vi "Table Size with and without Results.vi"(8 "error in":errorcluster, 9 "Table Configuration (Eingang)":T8 {"Cell Defaults"."Vertical Align" items=["Bottom", "Middle", "Top"]; "Cell Defaults"."Horizontal Align" items=["Center", "Justified", "JustifiedAll", "Left", "Right"]; "Table Settings"."Horizontal Align" items=["Center"=0, "Left"=3, "Right"=4]}, 11 "Table Content":T3={"TableHeader"=["Soll\nppm/%", "Ist\nppm/%", "Fehler\n%", "Toleranz\n%", "Ergebnis"], "Table"=[], "Relative Column Widths (%)"=[], "Results"={"Results"=[], "ResultPictures"={"Yes Ctl Refnum"=refnum, "No Ctl Refnum"=refnum}, "use Pictures"=FALSE, "Image Scale (%)"=100.0, "Autoscale? (T)"=TRUE, "Horizontal Align"=3, "Position"=0}, "PositionBemerkung"=enum."before", "PageBreak"=enum."before", "TablePictures"={"Ctl Refnum In"=[], "RowOrColumn"=enum."Row", "IndexToInsert"=0, "Image Scale (%)"=[], "Autoscale? (T)"=[], "Horizontal Align"=3}, "Horizontal Align"=3} {"Horizontal Align" items=["Center", "Justified", "JustifiedAll", "Left", "Right"]; "TablePictures"."Horizontal Align" items=["Center", "Justified", "JustifiedAll", "Left", "Right"]; "Results"."Position" items=["First", "Last"]; "Results"."Horizontal Align" items=["Center", "Justified", "JustifiedAll", "Left", "Right"]}) -> (0 "error out":errorcluster, 1 "Table Configuration (Ausgang)":T8 {"Cell Defaults"."Vertical Align" items=["Bottom", "Middle", "Top"]; "Cell Defaults"."Horizontal Align" items=["Center", "Justified", "JustifiedAll", "Left", "Right"]; "Table Settings"."Horizontal Align" items=["Center"=0, "Left"=3, "Right"=4]}, 2 "Table out":string[][](array[string]), 3 "Results out":T4={"Results"=[], "ResultPictures"={"Yes Ctl Refnum"=refnum, "No Ctl Refnum"=refnum}, "use Pictures"=FALSE, "Image Scale (%)"=100.0, "Autoscale? (T)"=TRUE, "Horizontal Align"=3, "Position"=0} {"Position" items=["First", "Last"]; "Horizontal Align" items=["Center", "Justified", "JustifiedAll", "Left", "Right"]}, 4 "Empty-Cluster":T1, 5 "TablePictures out":T2={"Ctl Refnum In"=[], "RowOrColumn"=enum."Row", "IndexToInsert"=0, "Image Scale (%)"=[], "Autoscale? (T)"=[], "Horizontal Align"=3} {"Horizontal Align" items=["Center", "Justified", "JustifiedAll", "Left", "Right"]}, 6 "TableHeader out":string[](array[string]), 7 "Horizontal Align":i32)   [LabVIEW 2020, in "PDF Interface.lvlib" / "PDF Interface Helper.lvlib"]
uses:
  PDF Interface Helper.lvlib
  <vilib>/Simplicity AI/SAI_PDF_API/Classes/Table Builder/Controls/SAI_PDF_Table Configuration.ctl
  <vilib>/Simplicity AI/SAI_PDF_API/Classes/Table Builder/Controls/SAI_PDF_Table Horizontal Align.ctl
  <vilib>/Simplicity AI/SAI_PDF_API/Classes/Table Builder/Controls/SAI_PDF_Default Cell Format.ctl
  <vilib>/Simplicity AI/SAI_PDF_API/Classes/Table Builder/Controls/SAI_PDF_BorderLine.ctl
  PDFResults.ctl
  PDFResultPictures.ctl
  PDFTableContentType.ctl
  PDFCommentPosition.ctl
  PDFPageBreak.ctl
  PDFTablePictures.ctl
  <vilib>/Simplicity AI/SAI_PDF_API/Classes/Table Builder/Table Builder.lvclass
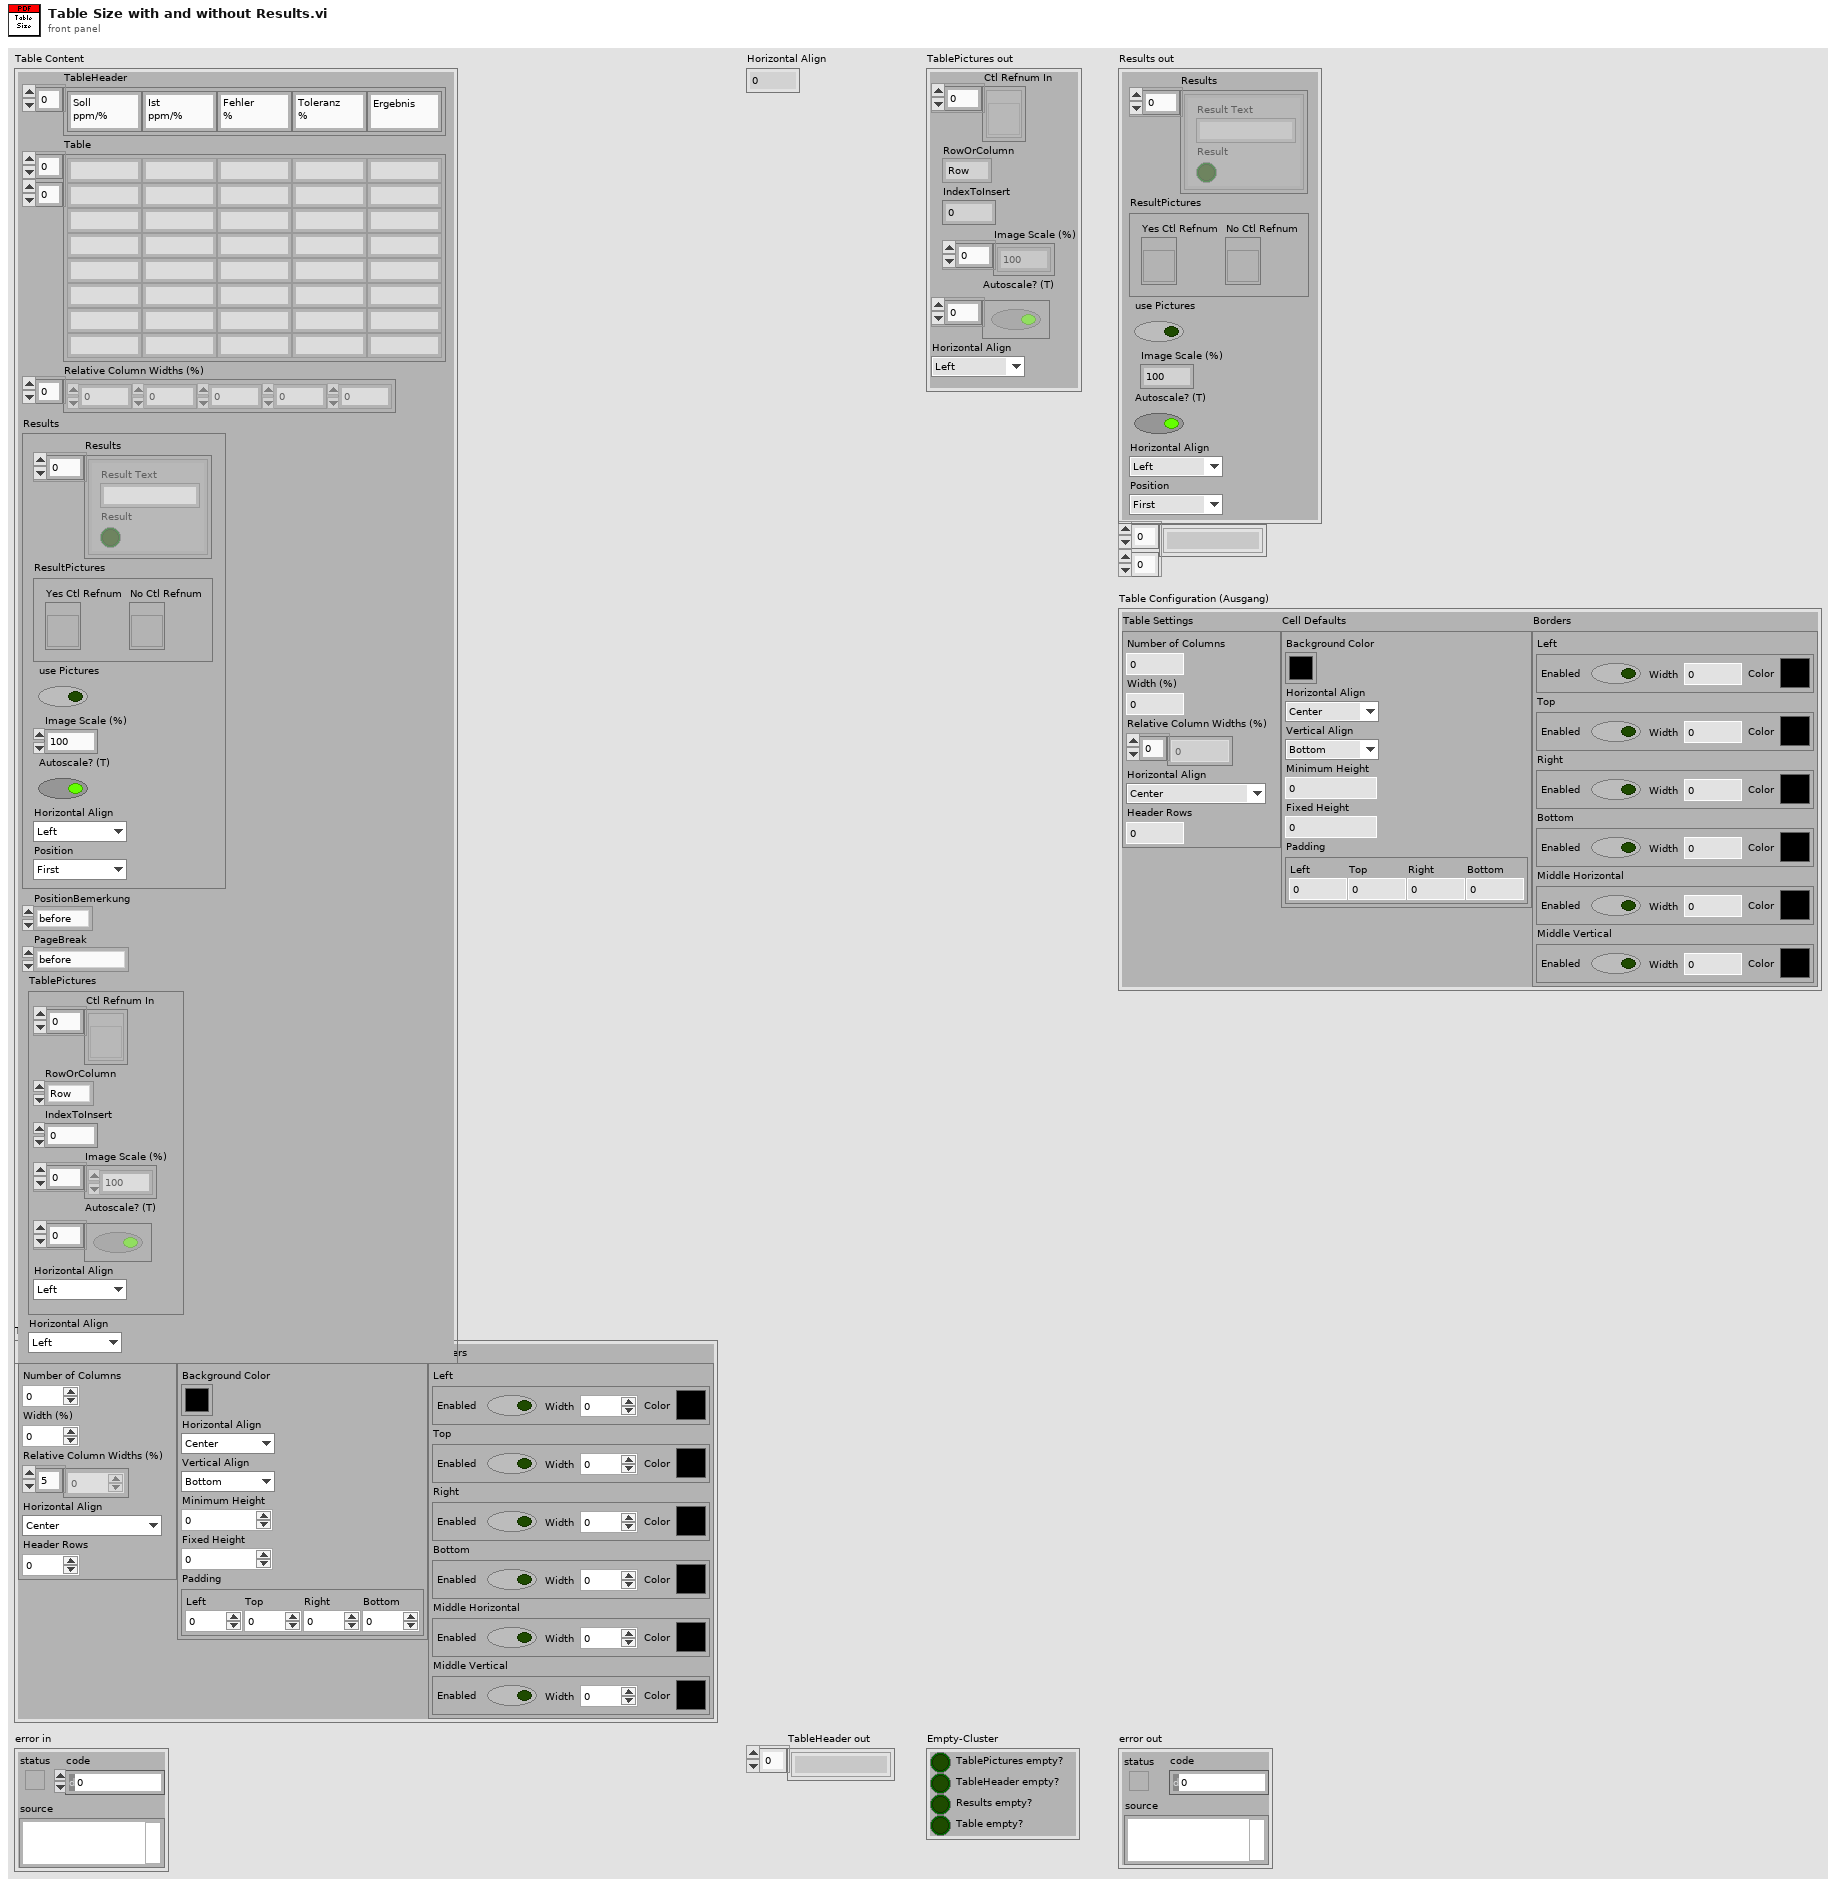
[diagram p1: front panel]
types:
  T1 = cluster{"TablePictures empty?":bool, "TableHeader empty?":bool, "Results empty?":bool, "Table empty?":bool}
  T2 = typedef "PDF Interface.lvlib/PDF Interface Helper.lvlib/PDFTablePictures.ctl" = cluster{"Ctl Refnum In":refnum<vi>[], "RowOrColumn":enum16{"Row", "Column"}, "IndexToInsert":u16, "Image Scale (%)":sgl[], "Autoscale? (T)":bool[], "Horizontal Align":i32}
  T3 = typedef "PDF Interface.lvlib/PDF Interface Helper.lvlib/PDFTableContentType.ctl" = cluster{"TableHeader":string[], "Table":string[][], "Relative Column Widths (%)":sgl[], "Results":T4, "PositionBemerkung":T6, "PageBreak":T7, "TablePictures":T2, "Horizontal Align":i32}
  T4 = typedef "PDF Interface.lvlib/PDF Interface Helper.lvlib/PDFResults.ctl" = cluster{"Results":cluster{"Result Text":string, "Result":bool}[], "ResultPictures":T5, "use Pictures":bool, "Image Scale (%)":sgl, "Autoscale? (T)":bool, "Horizontal Align":i32, "Position":i32}
  T5 = typedef "PDF Interface.lvlib/PDF Interface Helper.lvlib/PDFResultPictures.ctl" = cluster{"Yes Ctl Refnum":refnum<vi>, "No Ctl Refnum":refnum<vi>}
  T6 = typedef "PDF Interface.lvlib/PDF Interface Helper.lvlib/PDFCommentPosition.ctl" = enum16{"before", "after"}
  T7 = typedef "PDF Interface.lvlib/PDF Interface Helper.lvlib/PDFPageBreak.ctl" = enum16{"none", "before", "after", "after comment"}
  T8 = typedef "SAI_PDF_Toolkit.lvlib/Table Builder.lvclass/SAI_PDF_Table Configuration.ctl" = cluster{"Table Settings":cluster{"Number of Columns":i32, "Width (%)":sgl, "Relative Column Widths (%)":sgl[], "Horizontal Align":T9, "Header Rows":i32}, "Cell Defaults":T10, "Borders":cluster{"Left":T11, "Top":T11, "Right":T11, "Bottom":T11, "Middle Horizontal":T11, "Middle Vertical":T11}}
  T9 = typedef "SAI_PDF_Toolkit.lvlib/Table Builder.lvclass/SAI_PDF_Table Horizontal Align.ctl" = i32
  T10 = typedef "SAI_PDF_Toolkit.lvlib/Table Builder.lvclass/SAI_PDF_Default Cell Format.ctl" = cluster{"Background Color":u32, "Horizontal Align":i32, "Vertical Align":i32, "Minimum Height":sgl, "Fixed Height":sgl, "Padding":cluster{"Left":sgl, "Top":sgl, "Right":sgl, "Bottom":sgl}}
  T11 = typedef "SAI_PDF_Toolkit.lvlib/Table Builder.lvclass/SAI_PDF_BorderLine.ctl" = cluster{"Enabled":bool, "Width":sgl, "Color":u32}
  T12 = cluster{bool, "empty?":bool, "empty?":bool, bool}
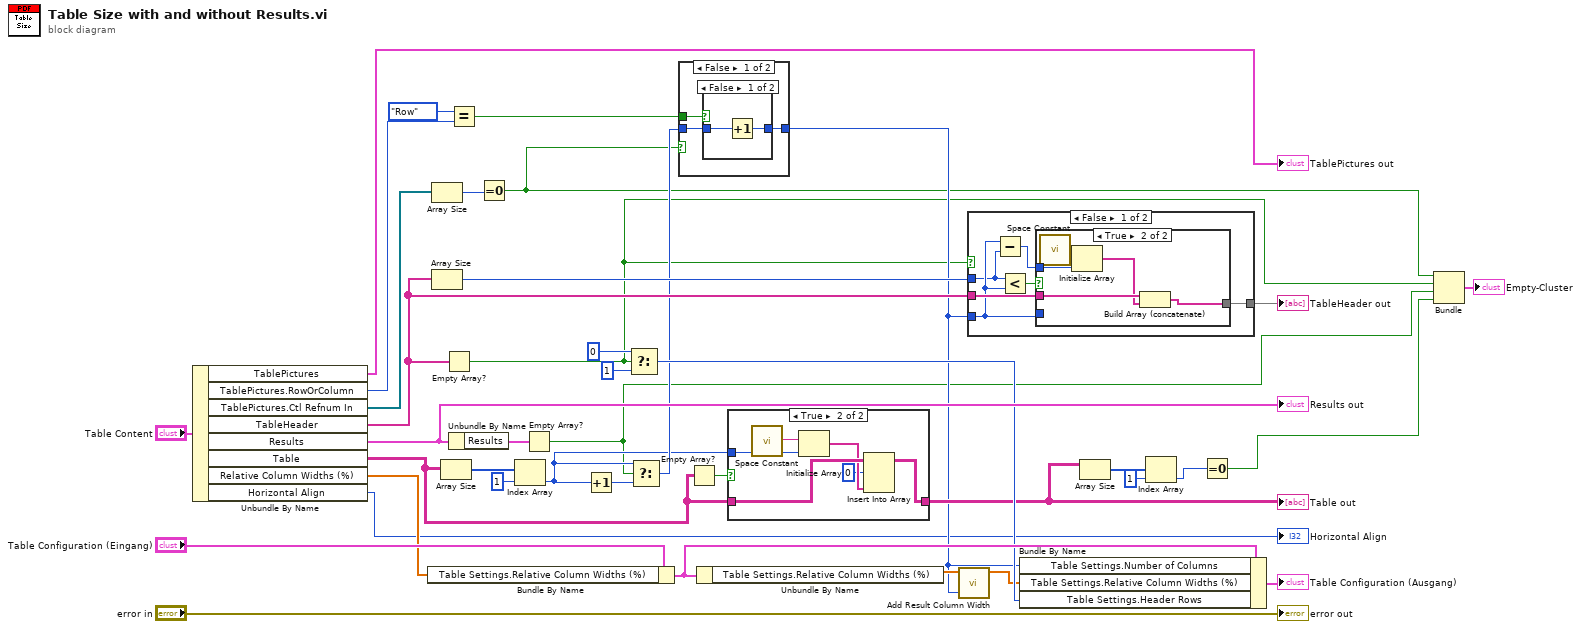
[diagram p0: block diagram]
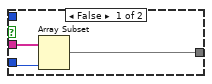
[diagram p5: hidden frame]
diagram:
  n1 = Unbundle By Name("Table Content") -> ("TablePictures"=→"TablePictures out":T2, "TablePictures.RowOrColumn"=w14:enum16{"Row", "Column"}, "TablePictures.Ctl Refnum In"=w16:refnum<vi>[], "TableHeader"=w26:string[], "Results"=w34:T4, "Table"=w23:string[][], "Relative Column Widths (%)"=w31:sgl[], "Horizontal Align"=→"Horizontal Align":i32)
  "Results out" <- w34
  n2 = Bundle By Name(cluster="Table Configuration (Eingang)", "Table Settings.Relative Column Widths (%)"=w31) -> (w32:T8)
  n3 = Array Size(array=w16) -> (size(s)=w15:i32)
  n4 = Array Size(array=w26) -> (size(s)=w27:i32)
  n5 = Array Size(array=w23) -> (size(s)=w38:i32[])
  n6 = Empty Array?(array=w26) -> (empty?=w7:bool)
  n7 = Equal?(x=enum16{"Row", "Column"}."Row", y=w14) -> (x = y?=w12:bool)
  n8 = Unbundle By Name(w34) -> ("Results"=w1:cluster{"Result Text":string, "Result":bool}[])
  n9 = Equal To 0?(x=w15) -> (x = 0?=w4:bool)
  n10 = Index Array(array=w38, index=1 ("Index")) -> (element=w9:i32)
  n11 = Empty Array?(array=w1) -> (empty?=w6:bool)
  n12 = Increment(x=w9) -> (x+1=w40:i32)
  n13 = Select(t=0, s=w7, f=1) -> (s? t:f=w28:i32)
  n14 = Select(t=w9, s=w6, f=w40) -> (s? t:f=w10:i32)
  n15 = case shown="False" w4 {
    tunnel: w12 -> [w43 _]
    tunnel: w10 -> [w42 w47]
    tunnel: [w41 w47] -> w11
    frame False {
      n16 = case shown="False" w43 {
        tunnel: w42 -> [w45 w46]
        tunnel: [w44 w46] -> w41
        frame False {
          n17 = Increment(x=w45) -> (x+1=w44:i32)
        }
        frame True {
        }
      }
    }
    frame True {
    }
  }
  n18 = Empty Array?(array=w23) -> (empty?=w24:bool)
  n19 = Unbundle By Name(w32) -> ("Table Settings.Relative Column Widths (%)"=w18:sgl[])
  n20 = case shown="True" w24 {
    tunnel: w23 -> [w48 w52]
    tunnel: [w48 w49] -> w22
    tunnel: w9 -> [_ w54]
    frame False {
    }
    frame True {
      n21 = call <vilib>:"Space Constant.vi"() -> ("String"=w53:string)
      n22 = Initialize Array(w53, w54) -> (w51:string[])
      n23 = Insert Into Array(array=w52, index (row)=0 ("Index (Zeile)"), new element=w51) -> (w49:string[][])  [unwired: 1 in]
    }
  }
  "Table out" <- w22
  n24 = call "Add Result Column Width.vi"("Result index"=w11, "Relative Column Widths (%)"=w18) -> ("Relative Column Widths (%) out"=w17:sgl[])  [unwired: 9 in]
  n25 = case shown="False" w7 {
    tunnel: w27 -> [w56 _]
    tunnel: w11 -> [w57 _]
    tunnel: w26 -> [w60 w69]
    tunnel: [w59 w69] -> w25
    frame False {
      n26 = Subtract(x=w57, y=w56) -> (x-y=w55:i32)
      n27 = Less?(x=w56, y=w57) -> (x < y?=w58:bool)
      n28 = case shown="True" w58 {
        tunnel: w60 -> [w63 w66]
        tunnel: [w62 w64] -> w59
        tunnel: w57 -> [w61 _]
        tunnel: w55 -> [_ w67]
        frame False {
          n29 = Array Subset(array=w63, length=w61) -> (w62:string[])  [unwired: 1 in]
        }
        frame True {
          n30 = call <vilib>:"Space Constant.vi"() -> ("String"=w68:string)
          n31 = Initialize Array(w68, w67) -> (w65:string[])
          n32 = Build Array (concatenate)(w66, w65) -> (w64:string[])
        }
      }
    }
    frame True {
    }
  }
  "TableHeader out" <- w25
  n33 = Bundle By Name(cluster=w32, "Table Settings.Number of Columns"=w11, "Table Settings.Relative Column Widths (%)"=w17, "Table Settings.Header Rows"=w28) -> (→"Table Configuration (Ausgang)":T8)
  n34 = Array Size(array=w22) -> (size(s)=w21:i32[])
  n35 = Index Array(array=w21, index=1 ("Index")) -> (element=w20:i32)
  n36 = Equal To 0?(x=w20) -> (x = 0?=w5:bool)
  n37 = Bundle(w4, "empty?"=w7, "empty?"=w6, w5) -> (→"Empty-Cluster":T12)  [unwired: 1 in]
  "error out" <- "error in"
